vi "Close.dyelaser.vi"(11 "DyeLaser":T1) -> ()   [LabVIEW 2022 SP3]
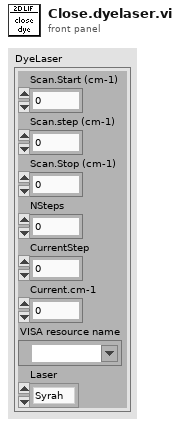
[diagram p1: front panel]
types:
  T1 = cluster{"Scan.Start (cm-1)":dbl, "Scan.Stop (cm-1)":dbl, "Scan.step (cm-1)":dbl, "VISA resource name":refnum<visa-resource-name>, "Laser":enum16{"Syrah", "Hyperdye"}, "NSteps":i32, "CurrentStep":i32, "Current.cm-1":dbl}
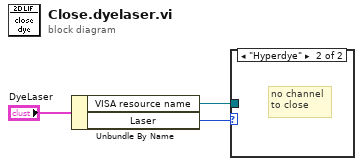
[diagram p0: block diagram]
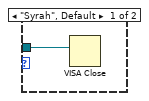
[diagram p2: hidden frame]
diagram:
  n1 = Unbundle By Name("DyeLaser") -> ("VISA resource name"=w3:refnum<visa-resource-name>, "Laser"=w1:enum16{"Syrah", "Hyperdye"})
  n2 = case shown="\"Hyperdye\"" w1 {
    tunnel: w3 -> [w4 _]
    frame "Syrah", Default {
      n3 = VISA Close(VISA resource name=w4) -> ()  [unwired: 1 in, 1 out]
    }
    frame "Hyperdye" {
      # "no channel\nto close"
    }
  }
